vi "FGV_SQL_EDITOR_records_display.vi"(4 "front_panel_reference":refnum<vi>, 6 "SQL_listbox_reference":refnum<vi>, 7 "options":T3, 8 "error_in":errorcluster, 11 "input":variant) -> (0 "error_out":errorcluster, 1 "all_info":T1, 2 "array_param_output":string[](array[string]), 3 "string_param_output":string)   [LabVIEW 2019]
uses:
  FGV_SQL_EDITOR_records_display.ctl
  SQL_EDITOR_all_info.ctl
  MAIN/SQL_record_states.ctl
  <userlib>/_OpenG.lib/array/array.llb/Filter 1D Array (String)__ogtk.vi
  <userlib>/_OpenG.lib/array/array.llb/Delete Elements from 1D Array (I32)__ogtk.vi
  <vilib>/addons/database/_DB Variant To Data/Database Variant To Data.xnode
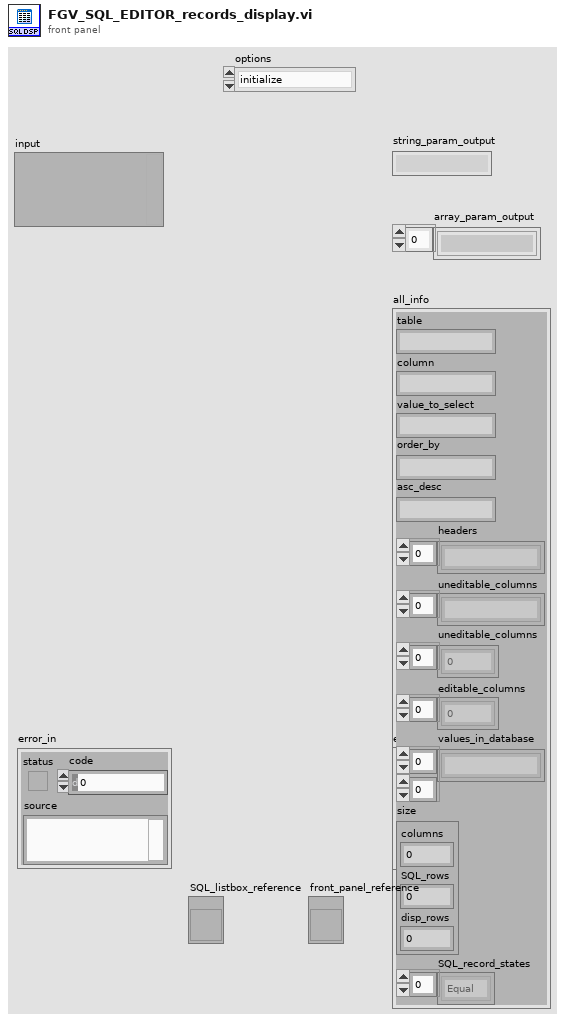
[diagram p1: front panel]
types:
  T1 = typedef "SQL_EDITOR_all_info.ctl" = cluster{"table":string, "column":string, "value_to_select":string, "order_by":string, "asc_desc":string, "headers":string[], "uneditable_columns":string[], "uneditable_columns":i32[], "editable_columns":i32[], "values_in_database":string[][], "size":cluster{"columns":i32, "SQL_rows":i32, "disp_rows":i32}, "SQL_record_states":T2[]}
  T2 = typedef "SQL_record_states.ctl" = enum16{"Equal", "Added", "Edited", "Deleted"}
  T3 = typedef "FGV_SQL_EDITOR_records_display.ctl" = enum16{"initialize", "set_table_name", "set_column_name", "set_value_to_select", "set_order_by", "set_asc_desc", "set_headers", "set_records", "get_table_name", "get_column_name", "get_value_to_select", "get_headers", "get_all_info", "record_added?", "record_inserted?", "record_edited?", "record_updated?", "record_deleted?", "discard_changes"}
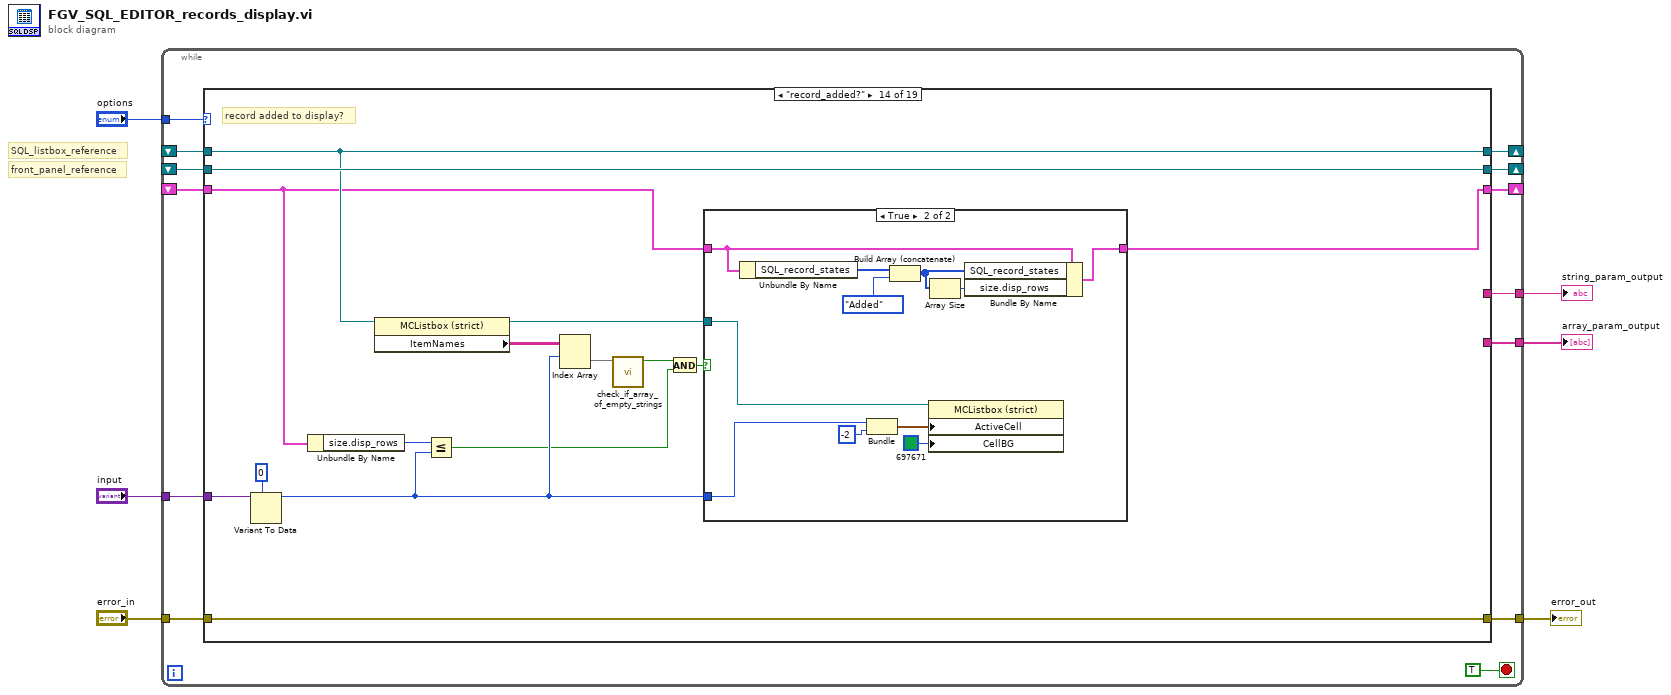
[diagram p0: block diagram]
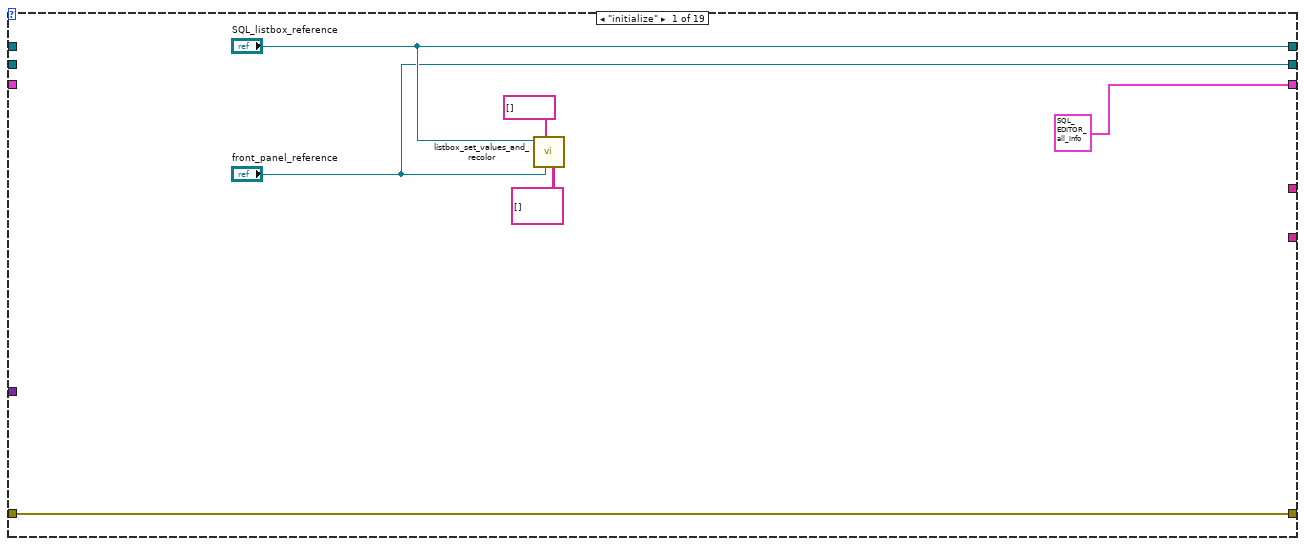
[diagram p2: hidden frame]
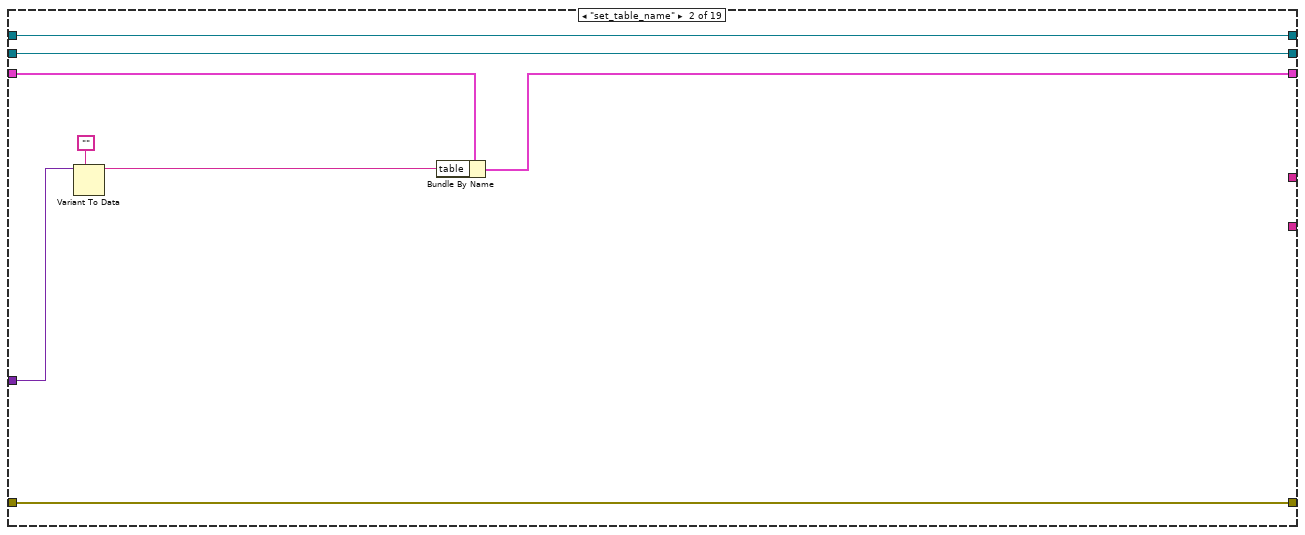
[diagram p3: hidden frame]
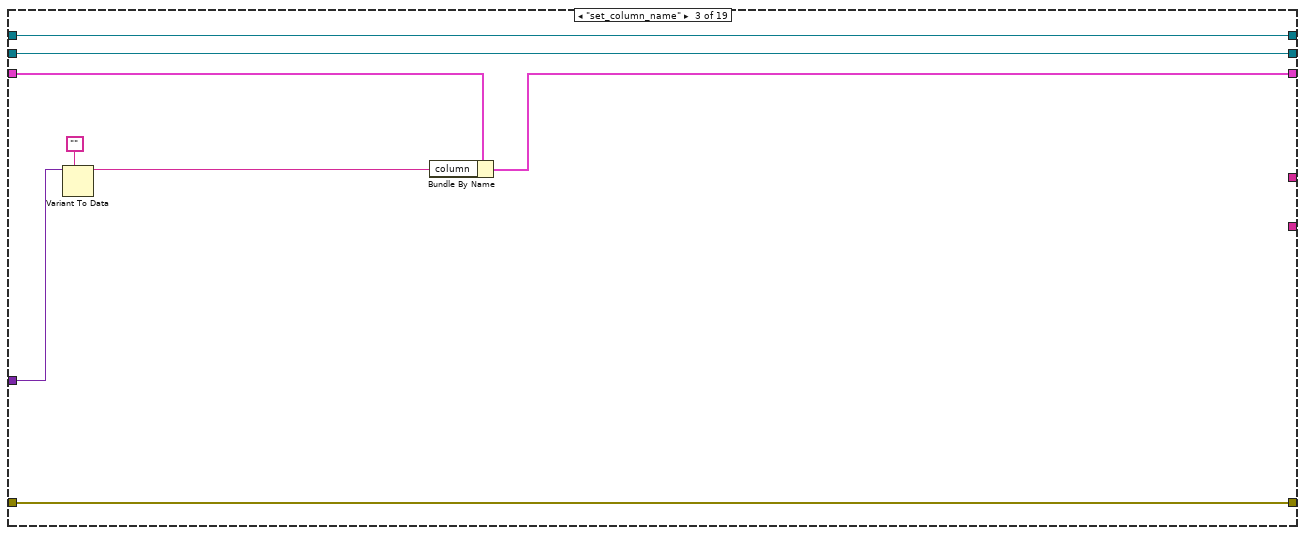
[diagram p4: hidden frame]
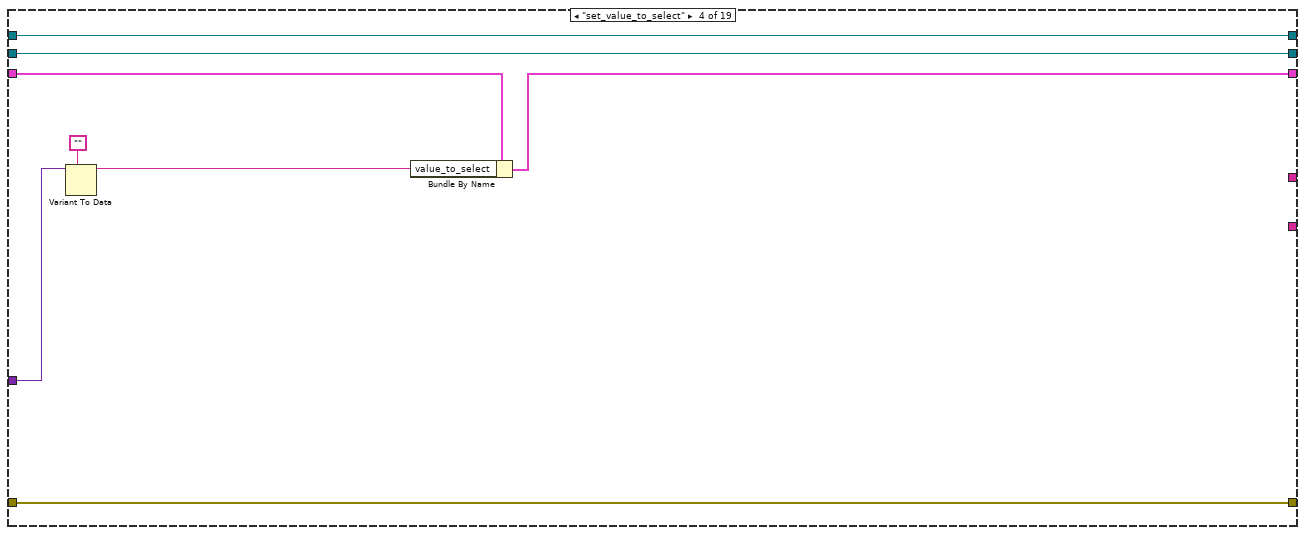
[diagram p5: hidden frame]
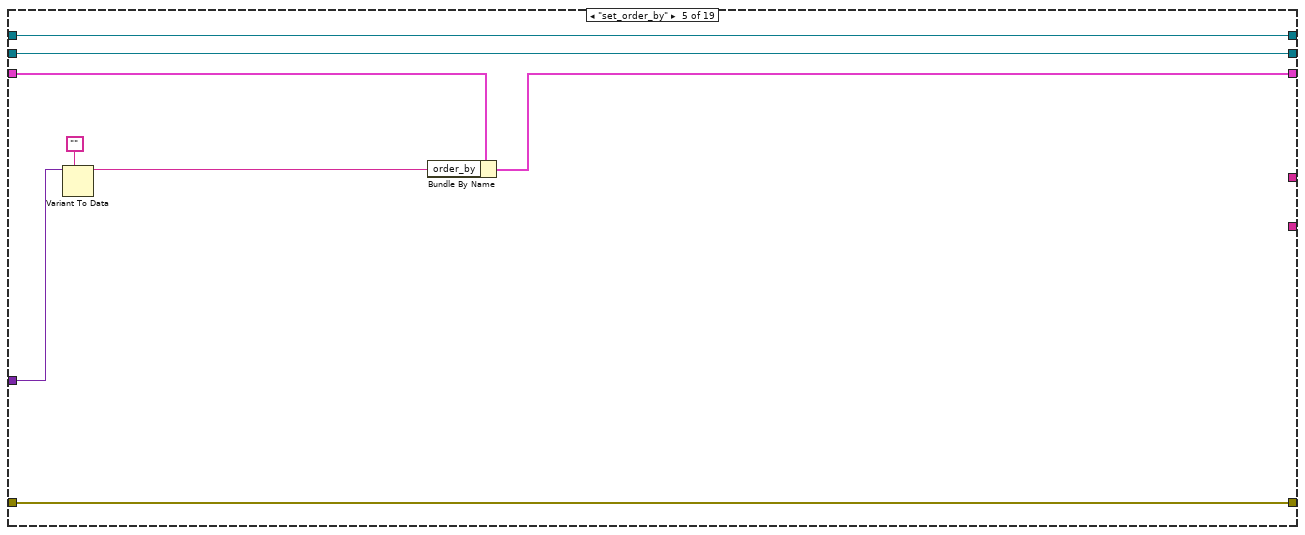
[diagram p6: hidden frame]
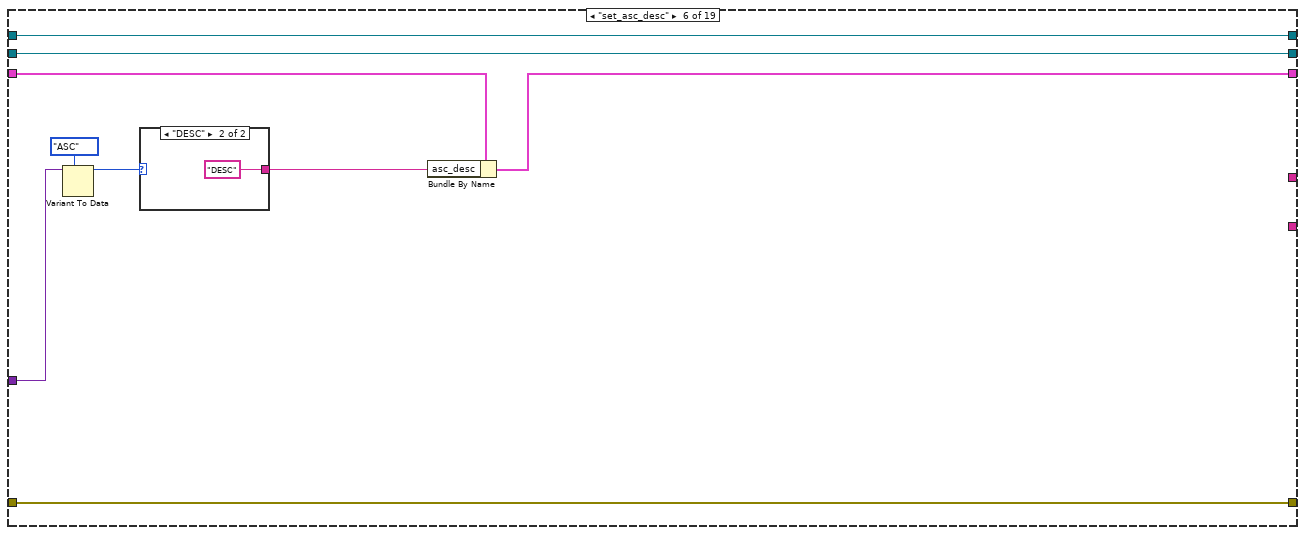
[diagram p7: hidden frame]
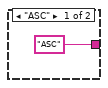
[diagram p8: hidden frame]
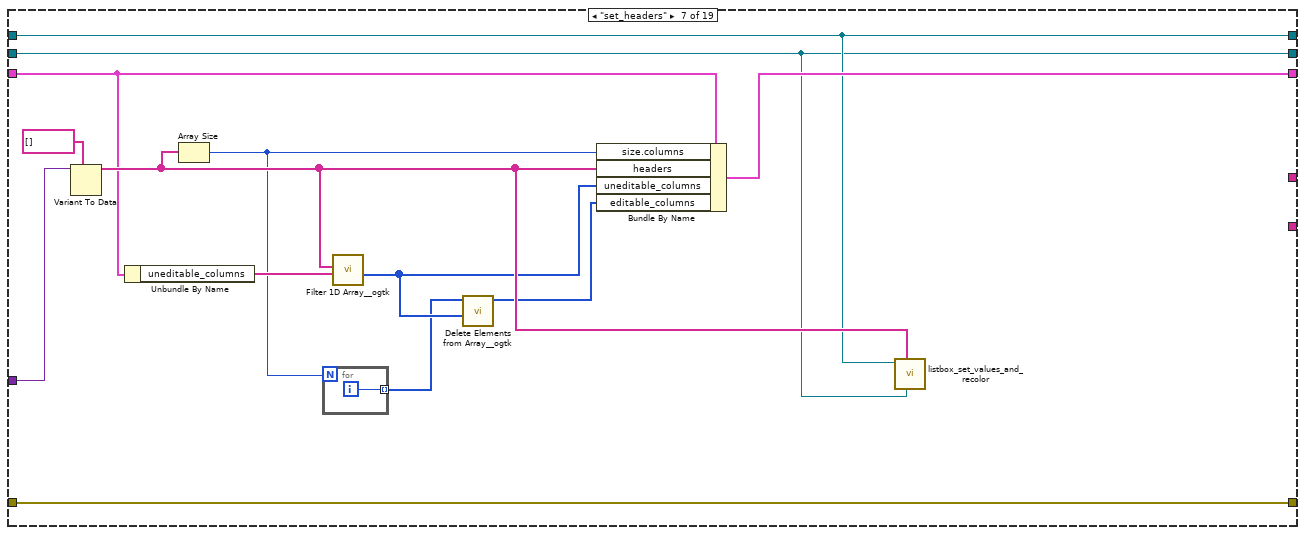
[diagram p9: hidden frame]
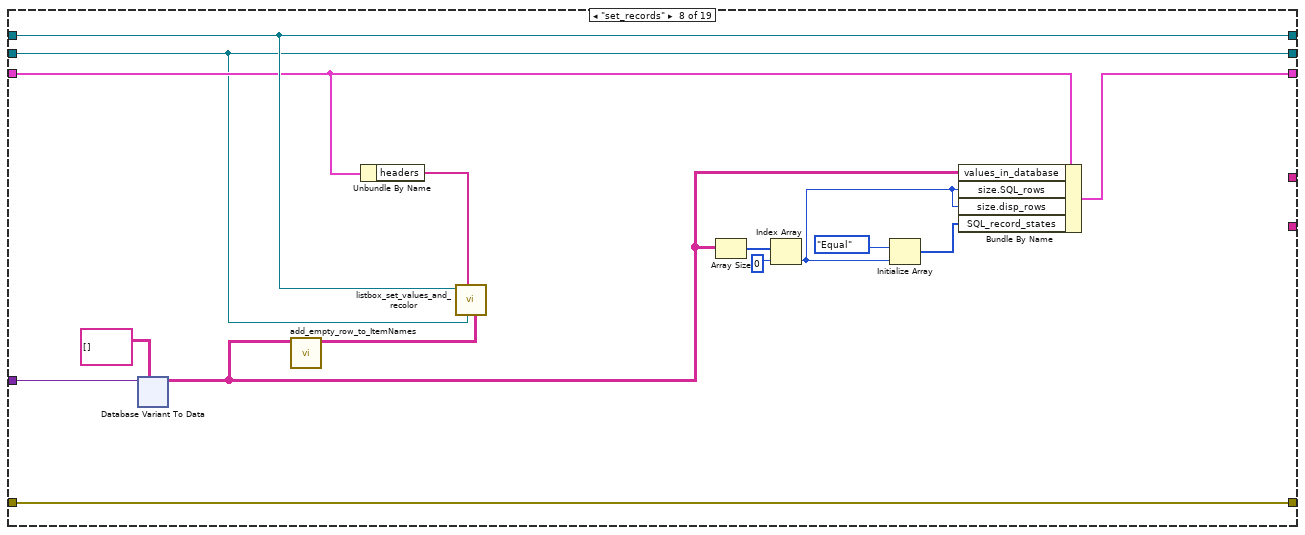
[diagram p10: hidden frame]
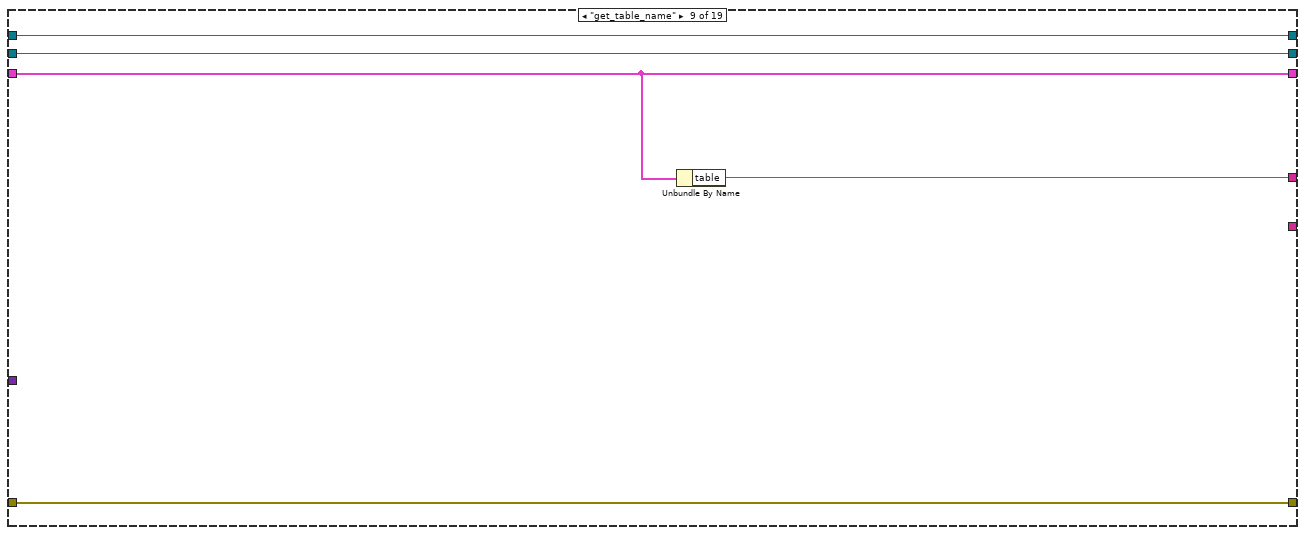
[diagram p11: hidden frame]
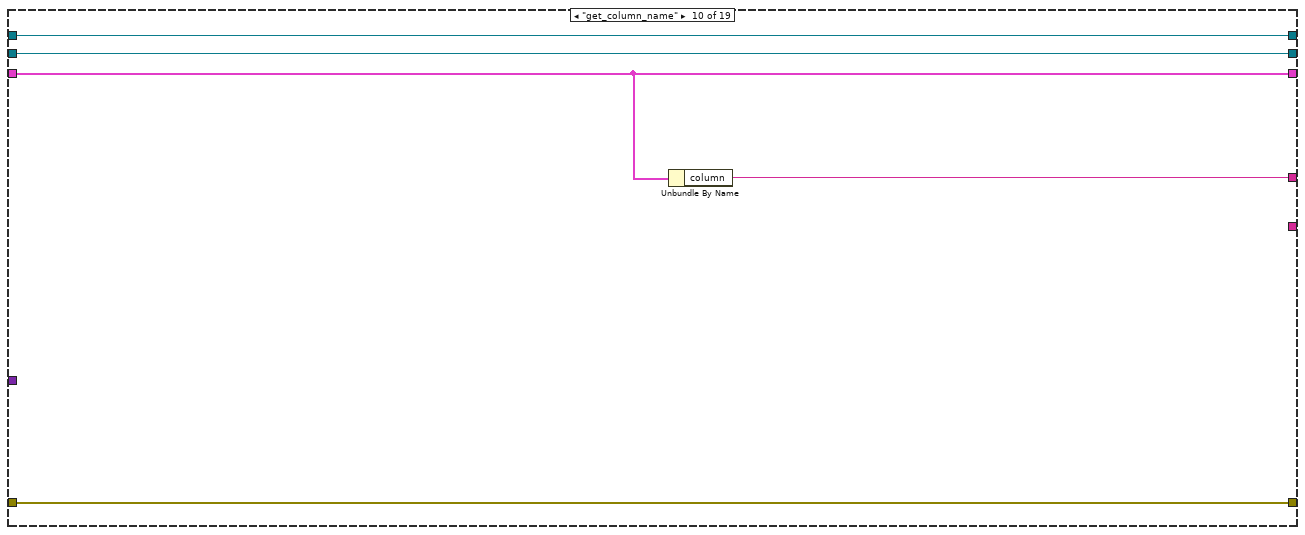
[diagram p12: hidden frame]
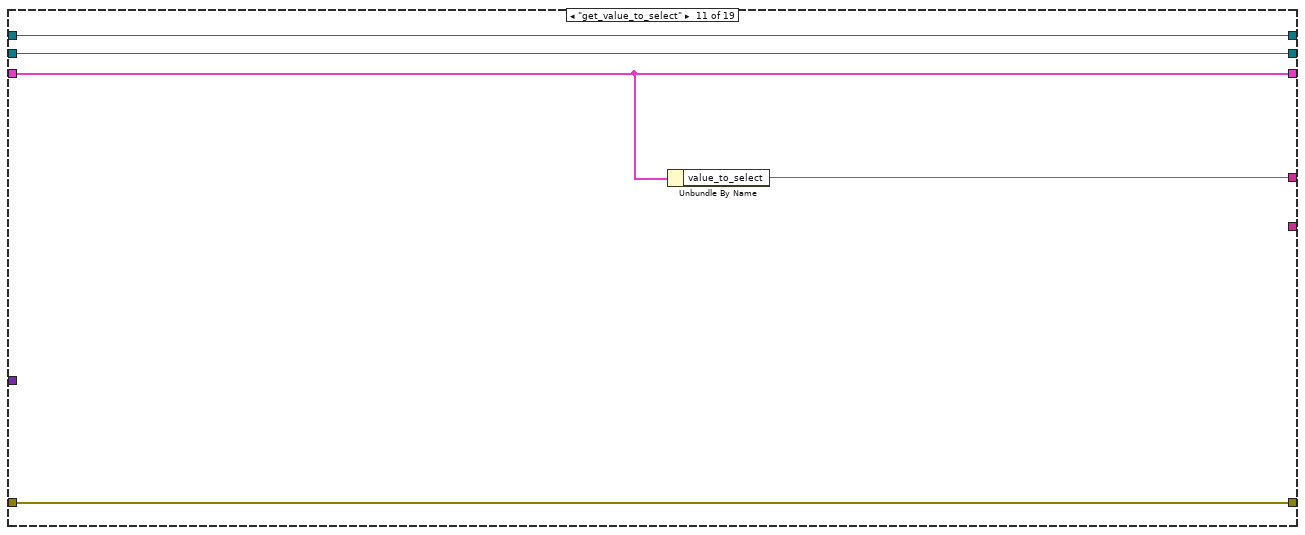
[diagram p13: hidden frame]
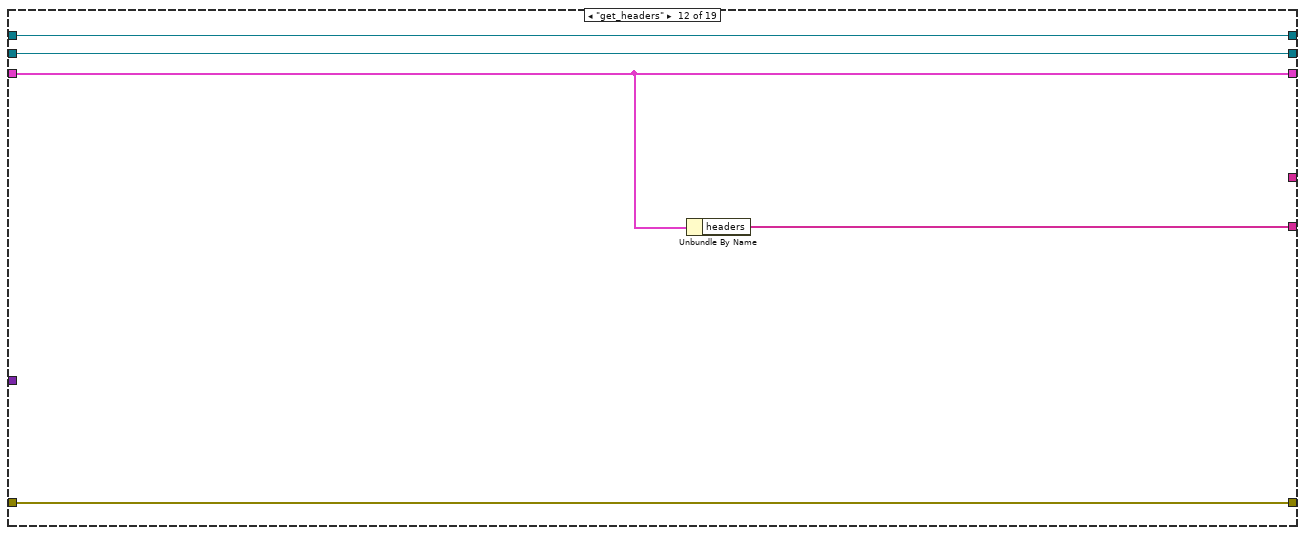
[diagram p14: hidden frame]
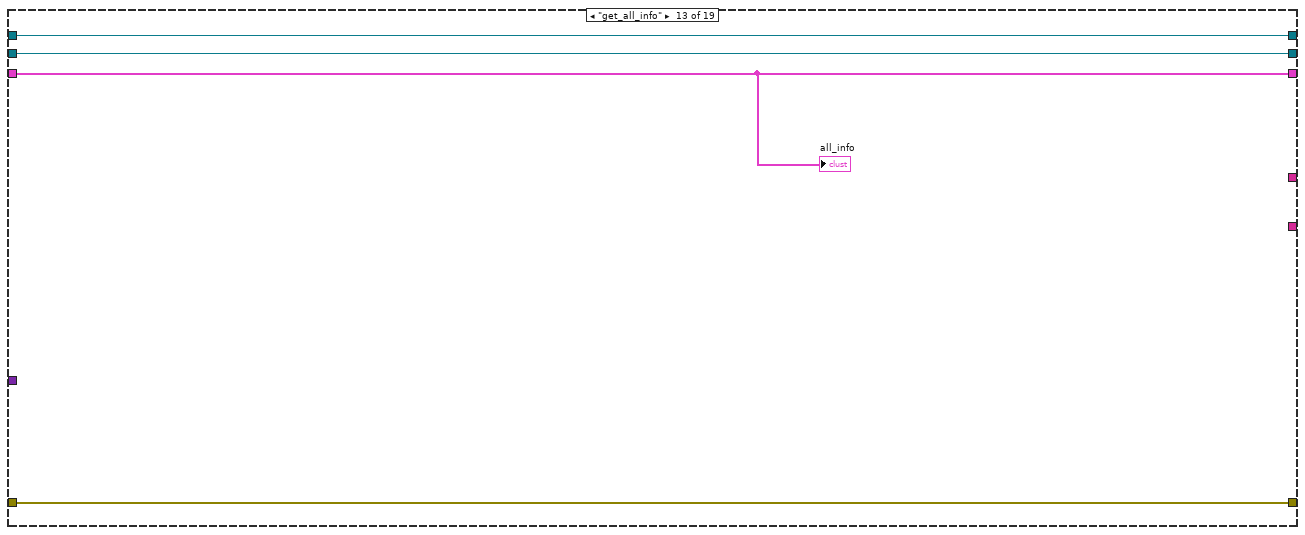
[diagram p15: hidden frame]
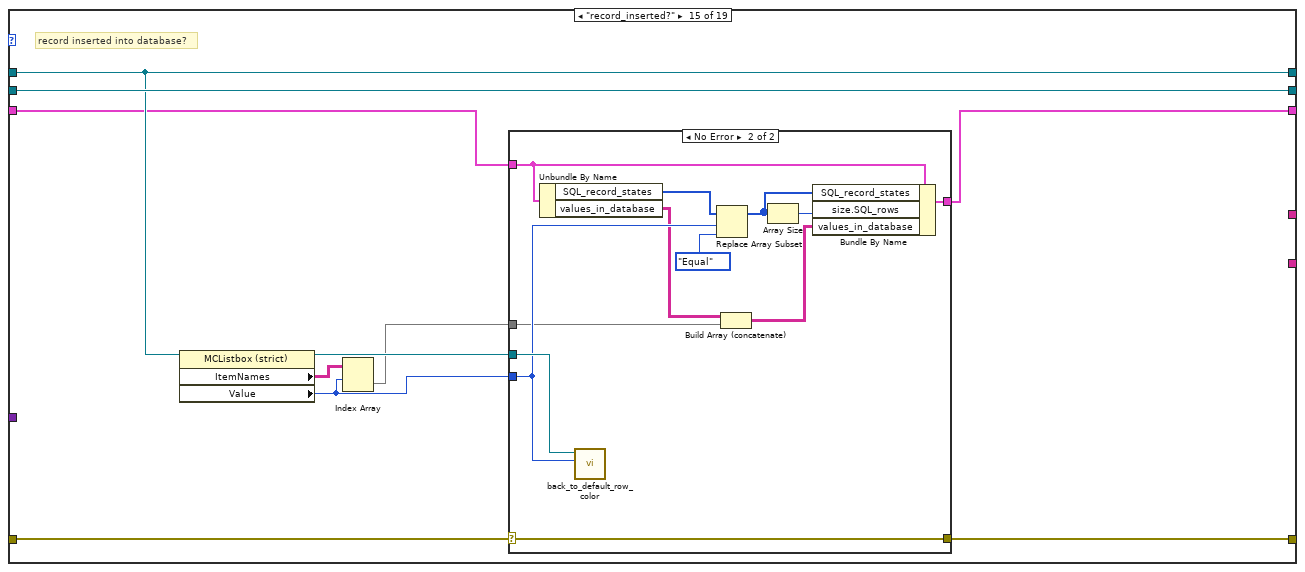
[diagram p17: hidden frame]
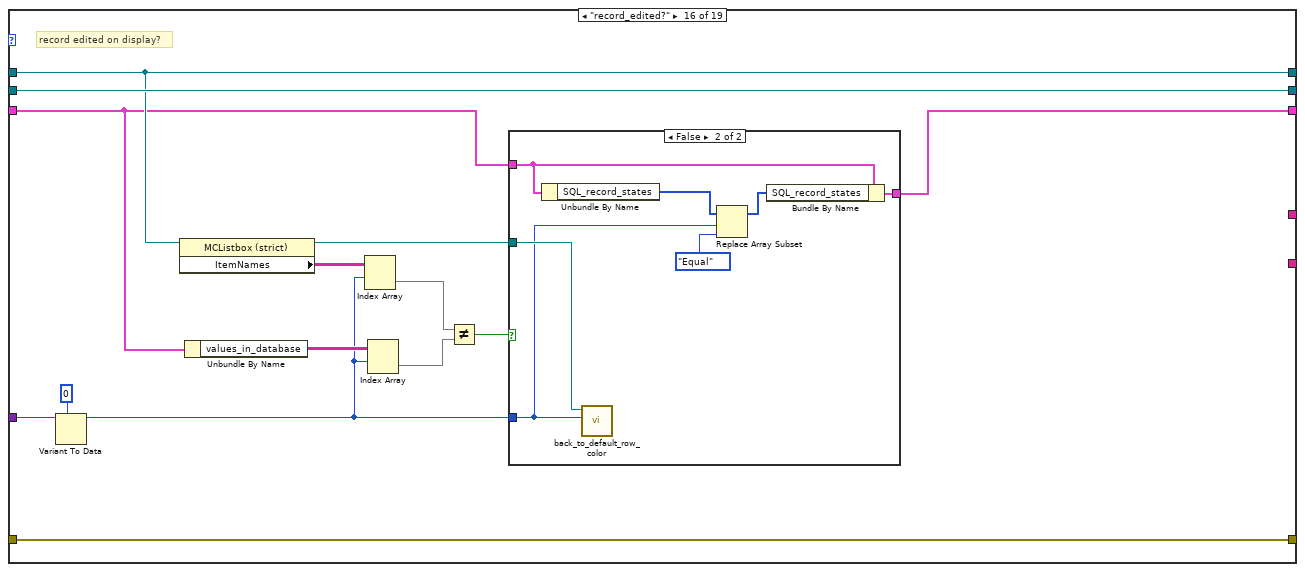
[diagram p19: hidden frame]
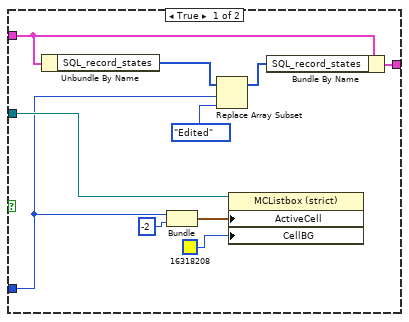
[diagram p20: hidden frame]
diagram:
  # "front_panel_reference"
  # "SQL_listbox_reference"
  n1 = while {
    tunnel: "options" -> [w18]
    tunnel: [w17] -> w6
    tunnel: "error_in" -> [w16]
    shift-right: [w15] -> _
    shift-left: _ -> [w14]
    tunnel: [w13] -> w3
    shift-right: [w12] -> _
    shift-left: _ -> [w11]
    tunnel: [w10] -> w2
    tunnel: "input" -> [w9]
    shift-right: [w8] -> _
    shift-left: _ -> [w7]
    stop <- TRUE stop-if-true
    n2 = case shown="\"record_added?\"" w18 {
      tunnel: [w25 w33 w41 w49 w57 w66 w81 w95 w132 w137 w142 w148 w152 w168 w184 w218 w239 w260 w285] -> w17
      tunnel: w16 -> [w25 w33 w41 w49 w57 w66 w81 w95 w132 w137 w142 w148 w152 w168 w185 w218 w240 w261 w285]
      tunnel: [T1 {"table"="", "column"="", "value_to_select"="", "order_by"="", "asc_desc"="", "headers"=[], "uneditable_columns"=[], "uneditable_columns"=[], "editable_columns"=[], "values_in_database"=[], "size"={"columns"=0, "SQL_rows"=0, "disp_rows"=0}, "SQL_record_states"=[]} ("SQL_selection") w31 w39 w47 w55 w64 w71 w91 w134 w139 w144 w149 w153 w161 w186 w205 w241 w262 w286] -> w15
      tunnel: w14 -> [_ w32 w40 w48 w56 w65 w72 w92 w134 w139 w144 w149 w153 w159 w187 w206 w242 w263 w281]
      tunnel: [_ _ _ _ _ _ _ _ w133 w138 w143 _ _ _ _ _ _ _ _] -> w13
      tunnel: ["SQL_listbox_reference" w30 w38 w46 w54 w63 w70 w94 w131 w136 w141 w147 w151 w164 w189 w213 w244 w265 w280] -> w12
      tunnel: w11 -> [_ w30 w38 w46 w54 w63 w70 w94 w131 w136 w141 w147 w151 w164 w189 w213 w244 w265 w280]
      tunnel: [_ _ _ _ _ _ _ _ _ _ _ w146 _ _ _ _ _ _ _] -> w10
      tunnel: w9 -> [_ w29 w36 w44 w52 w62 w73 w96 _ _ _ _ _ w166 _ w216 _ _ _]
      tunnel: ["front_panel_reference" w26 w34 w42 w50 w61 w69 w85 w130 w135 w140 w145 w150 w167 w190 w217 w245 w266 w288] -> w8
      tunnel: w7 -> [_ w26 w34 w42 w50 w61 w69 w85 w130 w135 w140 w145 w150 w167 w190 w217 w245 w266 w288]
      frame "initialize" {
        n3 = call "listbox_set_values_and_recolor.vi"("item_names"=string[][] [], "front_panel_reference"="front_panel_reference", "column_names"=string[] [], "multicolumn_listbox_reference_in"="SQL_listbox_reference") -> ()  [unwired: 6 in, 2 out]
      }
      frame "set_table_name" {
        n4 = Variant To Data(type="", Variant=w29) -> (data=w27:string)  [unwired: 1 in, 1 out]
        n5 = Bundle By Name(cluster=w32, "table"=w27) -> (w31:T1)
      }
      frame "set_column_name" {
        n6 = Variant To Data(type="", Variant=w36) -> (data=w35:string)  [unwired: 1 in, 1 out]
        n7 = Bundle By Name(cluster=w40, "column"=w35) -> (w39:T1)
      }
      frame "set_value_to_select" {
        n8 = Variant To Data(type="", Variant=w44) -> (data=w43:string)  [unwired: 1 in, 1 out]
        n9 = Bundle By Name(cluster=w48, "value_to_select"=w43) -> (w47:T1)
      }
      frame "set_order_by" {
        n10 = Variant To Data(type="", Variant=w52) -> (data=w51:string)  [unwired: 1 in, 1 out]
        n11 = Bundle By Name(cluster=w56, "order_by"=w51) -> (w55:T1)
      }
      frame "set_asc_desc" {
        n12 = Variant To Data(type=enum32{"ASC", "DESC"}."ASC" ("asc_desc"), Variant=w62) -> (data=w59:enum32{"ASC", "DESC"})  [unwired: 1 in, 1 out]
        n13 = case shown="\"DESC\"" w59 {
          tunnel: ["ASC" "DESC"] -> w58
          frame "ASC" {
          }
          frame "DESC" {
          }
        }
        n14 = Bundle By Name(cluster=w65, "asc_desc"=w58) -> (w64:T1)
      }
      frame "set_headers" {
        n15 = Variant To Data(type=string[] [], Variant=w73) -> (data=w79:string[])  [unwired: 1 in, 1 out]
        n16 = Unbundle By Name(w72) -> ("uneditable_columns"=w77:string[])
        n17 = Array Size(array=w79) -> (size(s)=w74:i32)
        n18 = for {
          N: w74 -> [_]
          tunnel: [w82] -> w76 mode=indexing
          i -> [w82]
        }
        n19 = call-poly <userlib>:"Filter 1D Array__ogtk.vi"("items to filter"=w77, "array"=w79) -> ("filtered item indices"=w78:i32[])  [unwired: 4 in, 1 out]
        n20 = call-poly <userlib>:"Delete Elements from Array__ogtk.vi"("indices"=w78, "array"=w76) -> ("array w/ subset deleted"=w75:i32[])  [unwired: 8 in, 1 out]
        n21 = Bundle By Name(cluster=w72, "size.columns"=w74, "headers"=w79, "uneditable_columns"=w78, "editable_columns"=w75) -> (w71:T1)
        n22 = call "listbox_set_values_and_recolor.vi"("front_panel_reference"=w69, "column_names"=w79, "multicolumn_listbox_reference_in"=w70) -> ()  [unwired: 7 in, 2 out]
      }
      frame "set_records" {
        n23 = xnode "Database Variant To Data"("database variant"=w96, "type"=string[][] []) -> ("data"=w83:string[][])  [unwired: 1 in, 1 out]
        n24 = call "add_empty_row_to_ItemNames.vi"("ItemNames_in"=w83) -> ("ItemNames_out"=w84:string[][])  [unwired: 10 in]
        n25 = Unbundle By Name(w92) -> ("headers"=w93:string[])
        n26 = call "listbox_set_values_and_recolor.vi"("item_names"=w84, "front_panel_reference"=w85, "column_names"=w93, "multicolumn_listbox_reference_in"=w94) -> ()  [unwired: 6 in, 2 out]
        n27 = Array Size(array=w83) -> (size(s)=w90:i32[])
        n28 = Index Array(array=w90, index=0) -> (element=w87:i32)
        n29 = Initialize Array(SQL_record_states."Equal", w87) -> (w86:T2[])
        n30 = Bundle By Name(cluster=w92, "values_in_database"=w83, "size.SQL_rows"=w87, "size.disp_rows"=w87, "SQL_record_states"=w86) -> (w91:T1)
      }
      frame "get_table_name" {
        n31 = Unbundle By Name(w134) -> ("table"=w133:string)
      }
      frame "get_column_name" {
        n32 = Unbundle By Name(w139) -> ("column"=w138:string)
      }
      frame "get_value_to_select" {
        n33 = Unbundle By Name(w144) -> ("value_to_select"=w143:string)
      }
      frame "get_headers" {
        n34 = Unbundle By Name(w149) -> ("headers"=w146:string[])
      }
      frame "get_all_info" {
        "all_info" <- w153
      }
      frame "record_added?" {
        # "record added to display?"
        n35 = Variant To Data(type=0, Variant=w166) -> (data=w157:i32)  [unwired: 1 in, 1 out]
        n36 = Unbundle By Name(w159) -> ("size.disp_rows"=w158:i32)
        n37 = property class="MCListbox (strict)"(reference=w164) -> (reference out=w162:refnum<vi>, "ItemNames"=w163:string[][])  [unwired: 1 in, 1 out]
        n38 = Less Or Equal?(x=w158, y=w157) -> (x <= y?=w156:bool)
        n39 = Index Array(array=w163, index (row)=w157) -> (element=w155:string[])  [unwired: 1 in]
        n40 = call "check_if_array_of_empty_strings.vi"("array"=w155) -> ("Not empty?"=w154:bool)  [unwired: 10 in]
        n41 = And(x=w154, y=w156) -> (x .and. y?=w160:bool)
        n42 = case shown="True" w160 {
          tunnel: w157 -> [_ w177]
          tunnel: w162 -> [_ w176]
          tunnel: w159 -> [w169 w174]
          tunnel: [w169 w175] -> w161
          frame False {
          }
          frame True {
            n43 = Unbundle By Name(w174) -> ("SQL_record_states"=w173:T2[])
            n44 = Bundle(w177, -2) -> (w178:cluster{i32, i32})  [unwired: 1 in]
            n45 = Build Array (concatenate)(w173, SQL_record_states."Added" ("new element/subarray")) -> (w171:T2[])
            n46 = property on="Property Node" class="MCListbox (strict)"(reference=w176, "ActiveCell"=w178, "CellBG"=u32 697671) -> ()  [unwired: 1 in, 2 out]
            n47 = Array Size(array=w171) -> (size(s)=w170:i32)
            n48 = Bundle By Name(cluster=w174, "SQL_record_states"=w171, "size.disp_rows"=w170) -> (w175:T1)
          }
        }
      }
      frame "record_inserted?" {
        # "record inserted into database?"
        n49 = property class="MCListbox (strict)"(reference=w189) -> (reference out=w188:refnum<vi>, "ItemNames"=w182:string[][], "Value"=w183:i32)  [unwired: 1 in, 1 out]
        n50 = Index Array(array=w182, index (row)=w183) -> (element=w181:string[])  [unwired: 1 in]
        n51 = case shown="No Error" w185 {
          selector: w185 -> [w192 w200]
          tunnel: w188 -> [_ w199]
          tunnel: w187 -> [w191 w202]
          tunnel: [w191 w201] -> w186
          tunnel: [w192 w200] -> w184
          tunnel: w183 -> [_ w198]
          tunnel: w181 -> [_ w196]
          frame Error {
          }
          frame No Error {
            n52 = Unbundle By Name(w202) -> ("SQL_record_states"=w203:T2[], "values_in_database"=w197:string[][])
            n53 = call "back_to_default_row_color.vi"("row"=w198, "listbox_reference"=w199) -> ()  [unwired: 9 in, 1 out]
            n54 = Replace Array Subset(array=w203, new element=SQL_record_states."Equal" ("new element/subarray"), index=w198) -> (w193:T2[])
            n55 = Build Array (concatenate)(w197, w196) -> (w195:string[][])
            n56 = Array Size(array=w193) -> (size(s)=w194:i32)
            n57 = Bundle By Name(cluster=w202, "SQL_record_states"=w193, "size.SQL_rows"=w194, "values_in_database"=w195) -> (w201:T1)
          }
        }
      }
      frame "record_edited?" {
        # "record edited on display?"
        n58 = Variant To Data(type=0, Variant=w216) -> (data=w207:i32)  [unwired: 1 in, 1 out]
        n59 = property class="MCListbox (strict)"(reference=w213) -> (reference out=w208:refnum<vi>, "ItemNames"=w212:string[][])  [unwired: 1 in, 1 out]
        n60 = Unbundle By Name(w206) -> ("values_in_database"=w214:string[][])
        n61 = Index Array(array=w212, index (row)=w207) -> (element=w211:string[])  [unwired: 1 in]
        n62 = Index Array(array=w214, index (row)=w207) -> (element=w210:string[])  [unwired: 1 in]
        n63 = Not Equal?(x=w211, y=w210) -> (x != y?=w209:bool)
        n64 = case shown="False" w209 {
          tunnel: w207 -> [w224 w229]
          tunnel: w208 -> [w226 w230]
          tunnel: w206 -> [w221 w233]
          tunnel: [w219 w231] -> w205
          frame True {
            n65 = Unbundle By Name(w221) -> ("SQL_record_states"=w222:T2[])
            n66 = Bundle(w224, -2) -> (w227:cluster{i32, i32})  [unwired: 1 in]
            n67 = Replace Array Subset(array=w222, new element=SQL_record_states."Edited" ("new element/subarray"), index=w224) -> (w220:T2[])
            n68 = property on="Property Node" class="MCListbox (strict)"(reference=w226, "ActiveCell"=w227, "CellBG"=u32 16318208) -> ()  [unwired: 1 in, 2 out]
            n69 = Bundle By Name(cluster=w221, "SQL_record_states"=w220) -> (w219:T1)
          }
          frame False {
            n70 = Unbundle By Name(w233) -> ("SQL_record_states"=w234:T2[])
            n71 = call "back_to_default_row_color.vi"("row"=w229, "listbox_reference"=w230) -> ()  [unwired: 9 in, 1 out]
            n72 = Replace Array Subset(array=w234, new element=SQL_record_states."Equal" ("new element/subarray"), index=w229) -> (w232:T2[])
            n73 = Bundle By Name(cluster=w233, "SQL_record_states"=w232) -> (w231:T1)
          }
        }
      }
      frame "record_updated?" {
        # "record updated in database?"
        n74 = property class="MCListbox (strict)"(reference=w244) -> (reference out=w243:refnum<vi>, "ItemNames"=w237:string[][], "Value"=w238:i32)  [unwired: 1 in, 1 out]
        n75 = Index Array(array=w237, index (row)=w238) -> (element=w236:string[])  [unwired: 1 in]
        n76 = case shown="No Error" w240 {
          selector: w240 -> [w247 w253]
          tunnel: w243 -> [_ w252]
          tunnel: w242 -> [w246 w256]
          tunnel: [w246 w254] -> w241
          tunnel: [w247 w253] -> w239
          tunnel: w238 -> [_ w248]
          tunnel: w236 -> [_ w249]
          frame Error {
          }
          frame No Error {
            n77 = Unbundle By Name(w256) -> ("SQL_record_states"=w257:T2[], "values_in_database"=w250:string[][])
            n78 = call "back_to_default_row_color.vi"("row"=w248, "listbox_reference"=w252) -> ()  [unwired: 9 in, 1 out]
            n79 = Replace Array Subset(array=w250, new element=w249, index (row)=w248) -> (w251:string[][])  [unwired: 1 in]
            n80 = Replace Array Subset(array=w257, new element=SQL_record_states."Equal" ("new element/subarray"), index=w248) -> (w255:T2[])
            n81 = Bundle By Name(cluster=w256, "SQL_record_states"=w255, "values_in_database"=w251) -> (w254:T1)
          }
        }
      }
      frame "record_deleted?" {
        # "record deleted from database?"
        n82 = property class="MCListbox (strict)"(reference=w265) -> (reference out=w264:refnum<vi>, "Value"=w259:i32)  [unwired: 1 in, 1 out]
        n83 = case shown="No Error" w261 {
          selector: w261 -> [w268 w269]
          tunnel: w264 -> [_ w277]
          tunnel: w263 -> [w267 w273]
          tunnel: [w267 w271] -> w262
          tunnel: [w268 w269] -> w260
          tunnel: w259 -> [_ w270]
          frame Error {
          }
          frame No Error {
            n84 = Unbundle By Name(w273) -> ("SQL_record_states"=w274:T2[])
            n85 = Bundle("Value"=w270, -2) -> (w278:cluster{"Value":i32, i32})  [unwired: 1 in]
            n86 = Replace Array Subset(array=w274, new element=SQL_record_states."Deleted" ("new element/subarray"), index=w270) -> (w272:T2[])
            n87 = property on="Property Node" class="MCListbox (strict)"(reference=w277, "ActiveCell"=w278, "CellBG"=u32 16711763) -> ()  [unwired: 1 in, 2 out]
            n88 = Bundle By Name(cluster=w273, "SQL_record_states"=w272) -> (w271:T1)
          }
        }
      }
      frame "discard_changes" {
        # "discard changes on display"
        n89 = property class="MCListbox (strict)"(reference=w280) -> (reference out=w287:refnum<vi>, "Value"=w283:i32)  [unwired: 1 in, 1 out]
        n90 = Unbundle By Name(w281) -> ("SQL_record_states"=w284:T2[])
        n91 = Index Array(array=w284, index=w283) -> (element=w282:T2)
        n92 = case shown="\"Added\"" w282 {
          tunnel: w287 -> [_ w303 w309]
          tunnel: w281 -> [w289 w302 w318]
          tunnel: [w289 w301 w317] -> w286
          tunnel: w283 -> [_ w293 w308]
          tunnel: w281 -> [_ w298 w316]
          tunnel: w280 -> [_ w296 w314]
          frame Default {
          }
          frame "Edited" {
            n93 = Unbundle By Name(w298) -> ("values_in_database"=w294:string[][], "SQL_record_states"=w297:T2[])
            n94 = property class="MCListbox (strict)"(reference=w296) -> (reference out=w291:refnum<vi>, "ItemNames"=w295:string[][])  [unwired: 1 in, 1 out]
            n95 = call "back_to_default_row_color.vi"("row"=w293, "listbox_reference"=w303) -> ()  [unwired: 9 in, 1 out]
            n96 = Index Array(array=w294, index (row)=w293) -> (element=w292:string[])  [unwired: 1 in]
            n97 = Replace Array Subset(array=w297, new element=SQL_record_states."Equal" ("new element/subarray"), index=w293) -> (w299:T2[])
            n98 = Replace Array Subset(array=w295, new element=w292, index (row)=w293) -> (w290:string[][])  [unwired: 1 in]
            n99 = property class="MCListbox (strict)"(reference=w291, "ItemNames"=w290) -> ()  [unwired: 1 in, 2 out]
            n100 = Bundle By Name(cluster=w302, "SQL_record_states"=w299) -> (w301:T1)
          }
          frame "Added" {
            n101 = property class="MCListbox (strict)"(reference=w314) -> (reference out=w304:refnum<vi>, "ItemNames"=w313:string[][])  [unwired: 1 in, 1 out]
            n102 = Unbundle By Name(w316) -> ("SQL_record_states"=w315:T2[])
            n103 = Bundle("Value"=w308, -2) -> (w312:cluster{"Value":i32, i32})  [unwired: 1 in]
            n104 = property on="Property Node" class="MCListbox (strict)"(reference=w309, "ActiveCell"=w312, "CellBG"=u32 16448250) -> ()  [unwired: 1 in, 2 out]
            n105 = Delete From Array(array=w315, index=w308) -> (array with subset deleted=w306:T2[])  [unwired: 1 in, 1 out]
            n106 = Delete From Array(array=w313, index (row)=w308) -> (array with subset deleted=w305:string[][])  [unwired: 2 in, 1 out]
            n107 = Array Size(array=w306) -> (size(s)=w307:i32)
            n108 = call "add_empty_row_to_ItemNames.vi"("multicolumn_listbox_reference_in"=w304, "ItemNames_in"=w305) -> ()  [unwired: 9 in, 1 out]
            n109 = Bundle By Name(cluster=w318, "size.disp_rows"=w307, "SQL_record_states"=w306) -> (w317:T1)
          }
        }
      }
    }
  }
  "error_out" <- w6
  "string_param_output" <- w3
  "array_param_output" <- w2
